vi "1_Addition of two nos.vi"() -> ()   [LabVIEW 2018]
panel:
  out "Output No.-":dbl
  in  "Second No.-":i16
  in  "First No.-":i32
  # "Develop HMI to add two numbers"
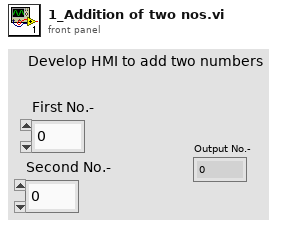
[diagram p1: front panel]
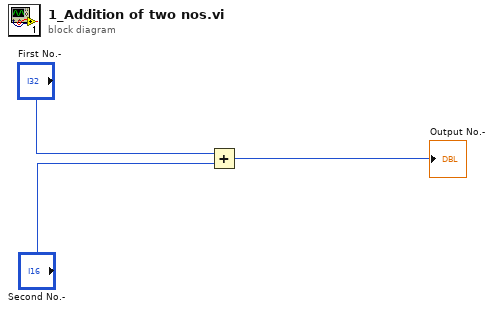
[diagram p0: block diagram]
diagram:
  n1 = Add(x="First No.-", y="Second No.-") -> (x+y=→"Output No.-":i32)
